vi "dlgSelectVisApps.vi"(8 "Error In":errorcluster[](array[cluster]), 10 "PathsToVisApps":string[](array[string])=["VisualizeStatus", "VisualizeWfrm", "VisualizeAnalysis"]) -> (0 "Error Out":errorcluster[](array[cluster]))   [LabVIEW 2018, in "Visualization.lvlib"]
uses:
  Visualization.lvlib
  <userlib>/NIST/NISTErrorLib/NISTErrorLib.lvlib
panel:
  in  "btnCancel":bool
  in  "btnRun":bool
  in  "selArray":cluster{"chkSelect":bool, "strVis":string}[](array[cluster]) caption="Select Visualization Apps"
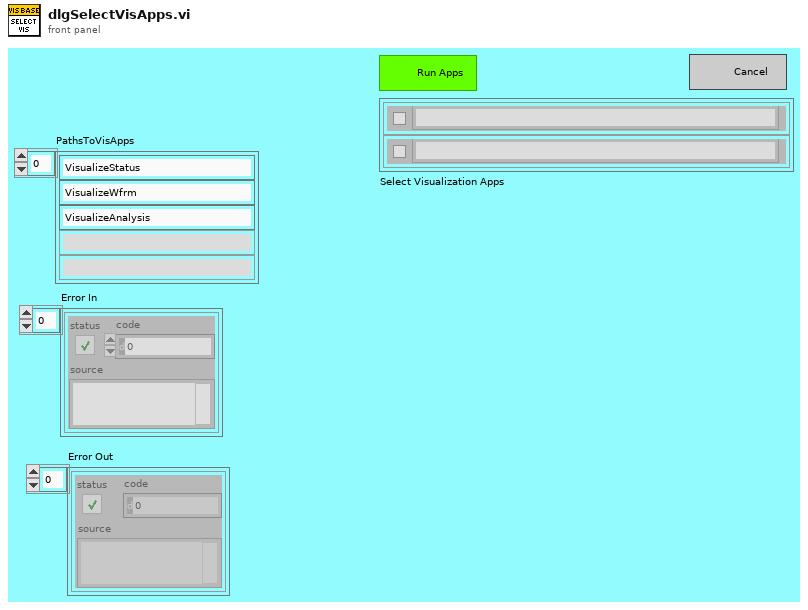
[diagram p1: front panel]
types:
  T1 = enum32{"Invalid", "Default", "Floating", "Floating/Auto-Hide", "Modal"}
  T2 = typedef "LVRectTypeDef.ctl" = cluster{"Left":i16, "Top":i16, "Right":i16, "Bottom":i16}
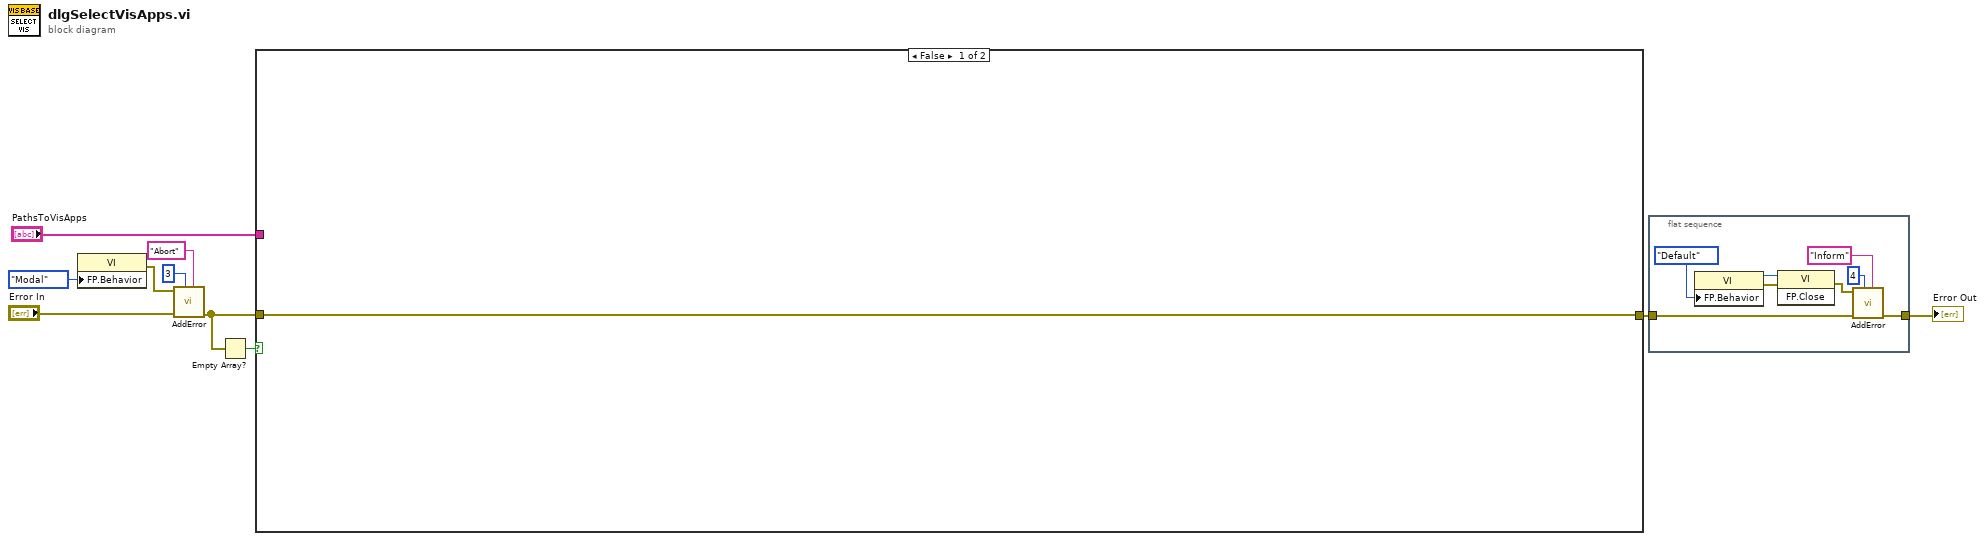
[diagram p0: block diagram]
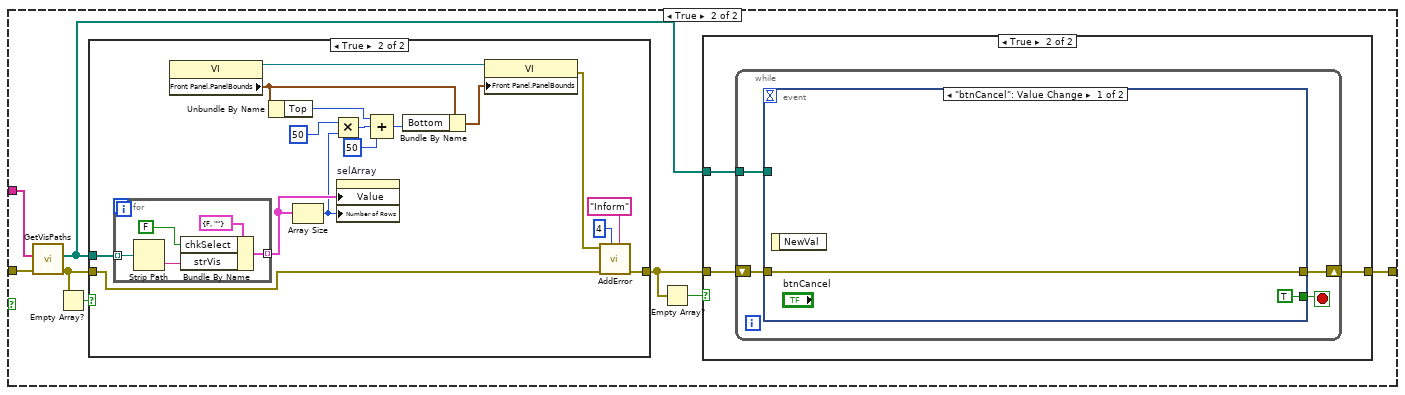
[diagram p2: hidden frame]
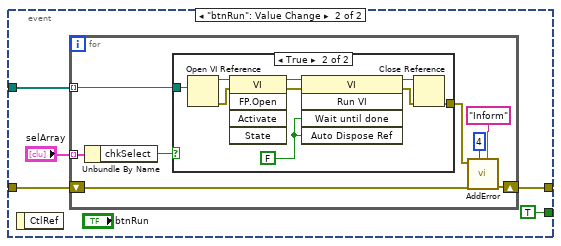
[diagram p4: hidden frame]
diagram:
  n1 = property class="VI"("FP.Behavior"=T1."Modal" ("Front Panel Window:Behavior")) -> (error out=w8:errorcluster)  [unwired: 2 in, 1 out]
  n2 = call <userlib>:"AddError.vi"("Severity"="Abort", "Priority"=u8 3, "ErrorArray"="Error In", "error in (no error)"=w8) -> ("ErrorArray"=w4:errorcluster[])  [unwired: 6 in, 1 out]
  n3 = Empty Array?(array=w4) -> (empty?=w5:bool)
  n4 = case shown="False" w5 {
    tunnel: w4 -> [w11 w19]
    tunnel: "PathsToVisApps" -> [_ w18]
    tunnel: [w11 w12] -> w2
    frame False {
    }
    frame True {
      n5 = call "GetVisPaths.vi"("ErrorArray in"=w19, "PathsToVisApps"=w18) -> ("ErrorArray out"=w17:errorcluster[], "VisPaths"=w13:path[])  [unwired: 8 in]
      n6 = Empty Array?(array=w17) -> (empty?=w16:bool)
      n7 = case shown="True" w16 {
        tunnel: w13 -> [_ w68]
        tunnel: w17 -> [w52 w57]
        tunnel: [w52 w56] -> w14
        frame False {
        }
        frame True {
          n8 = for {
            tunnel: w68 -> [w72] mode=indexing
            tunnel: [w69] -> w67 mode=indexing
            n9 = Strip Path(path=w72) -> (name=w71:string)  [unwired: 1 out]
            n10 = Bundle By Name(cluster=cluster{"chkSelect":bool, "strVis":string} {"chkSelect"=FALSE, "strVis"=""} ("elementSelArray"), "chkSelect"=FALSE, "strVis"=w71) -> (w69:cluster{"chkSelect":bool, "strVis":string})
          }
          n11 = property class="VI"() -> (reference out=w59:refnum<vi>, "Front Panel.PanelBounds"=w62:T2)  [unwired: 2 in, 1 out]
          n12 = Unbundle By Name(w62) -> ("Top"=w63:i16)
          n13 = Array Size(array=w67) -> (size(s)=w66:i32)
          n14 = Multiply(x=50, y=w66) -> (x*y=w64:i32)
          n15 = property on="selArray" class="Arr (strict)"("Value"=w67, "Number of Rows"=w66) -> ()  [unwired: 2 in, 2 out]
          n16 = Compound Arithmetic op=ADD(w63, w64, 50 ("value")) -> (w61:i32)
          n17 = Bundle By Name(cluster=w62, "Bottom"=w61) -> (w60:T2)
          n18 = property class="VI"(reference=w59, "Front Panel.PanelBounds"=w60) -> (error out=w55:errorcluster)  [unwired: 1 in, 1 out]
          n19 = call <userlib>:"AddError.vi"("Severity"="Inform", "Priority"=u8 4, "ErrorArray"=w57, "error in (no error)"=w55) -> ("ErrorArray"=w56:errorcluster[])  [unwired: 6 in, 1 out]
        }
      }
      n20 = Empty Array?(array=w14) -> (empty?=w15:bool)
      n21 = case shown="True" w15 {
        tunnel: w14 -> [w20 w23]
        tunnel: w13 -> [_ w22]
        tunnel: [w20 w21] -> w12
        frame False {
        }
        frame True {
          n22 = while {
            shift-right: [w25] -> w21
            shift-left: w23 -> [w26]
            tunnel: w22 -> [w24]
            stop <- w27 stop-if-true
            n23 = event shown="[0] \"btnCancel\": Value Change" {
              selector: _ -> [_ _]
              dyn-events: _ -> [_ _]
              timeout: _ -> [_ _]
              tunnel: [TRUE TRUE] -> w27
              tunnel: [w28 w30] -> w25
              tunnel: w26 -> [w28 w33]
              tunnel: w24 -> [_ w32]
              event "btnCancel": Value Change {
                n24 = event-data() -> ()  [unwired: 1 in, 1 out]
              }
              event "btnRun": Value Change {
                n25 = event-data() -> ()  [unwired: 1 in, 1 out]
                n26 = for {
                  tunnel: "selArray" -> [w42] mode=indexing
                  shift-right: [w39] -> w30
                  shift-left: w33 -> [w38]
                  tunnel: w32 -> [w40] mode=indexing
                  n27 = Unbundle By Name(w42) -> ("chkSelect"=w41:bool)
                  n28 = case shown="True" w41 {
                    tunnel: w40 -> [_ w51]
                    tunnel: [_ w43] -> w37
                    frame False {
                    }
                    frame True {
                      w48 = FALSE ("Wait Until Done")
                      n29 = Open VI Reference(vi path=w51) -> (vi reference=w50:refnum<vi>, error out=w45:errorcluster)  [unwired: 5 in]
                      n30 = invoke class="VI" method="FP.Open"(reference=w50, error in=w45) -> (reference out=w49:refnum<vi>, error out=w44:errorcluster)  [unwired: 3 in, 3 out]
                      n31 = invoke class="VI" method="Run VI"(reference=w49, error in=w44, "Wait until done"=w48, "Auto Dispose Ref"=w48) -> (reference out=w46:refnum<vi>, error out=w47:errorcluster)  [unwired: 1 in, 3 out]
                      n32 = Close Reference(reference=w46, error in (no error)=w47) -> (error out=w43:errorcluster)
                    }
                  }
                  n33 = call <userlib>:"AddError.vi"("Severity"="Inform", "Priority"=u8 4, "ErrorArray"=w38, "error in (no error)"=w37) -> ("ErrorArray"=w39:errorcluster[])  [unwired: 6 in, 1 out]
                }
              }
            }
          }
        }
      }
    }
  }
  n34 = flat-sequence {
    tunnel: w2 -> [w78]
    tunnel: [w74] -> w1
    frame #0 {
      n35 = property class="VI"("FP.Behavior"=T1."Default" ("Front Panel Window:Behavior")) -> (reference out=w80:refnum<vi>, error out=w79:errorcluster)  [unwired: 2 in]
      n36 = invoke class="VI" method="FP.Close"(reference=w80, error in=w79) -> (error out=w77:errorcluster)  [unwired: 1 in, 2 out]
      n37 = call <userlib>:"AddError.vi"("Severity"="Inform", "Priority"=u8 4, "ErrorArray"=w78, "error in (no error)"=w77) -> ("ErrorArray"=w74:errorcluster[])  [unwired: 6 in, 1 out]
    }
  }
  "Error Out" <- w1
